vi "探头温度系数.vi"(7 "校准参数":u16(ring) caption="校准参数：" items=["pH", "DO", "浊度", "电导率", "叶绿素a", "藻密度", "ORP", "DO2", "氯化物", "悬浮物"], 8 "error in (no error)":errorcluster caption="错误输入（无错误）", 11 "温度系数":dbl=25.0 caption="温度系数：" format="%#_6f") -> (0 "error out":errorcluster caption="错误输出")   [LabVIEW 2016, in "斯坦道多参数.lvlib"]
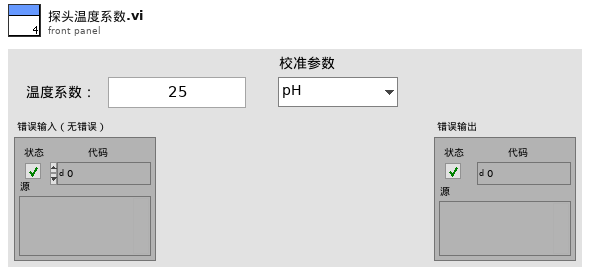
[diagram p1: front panel]
types:
  T1 = typedef "斯坦道多参数.lvlib/探头类型.ctl" = enum16{"禹山", "国弘", "纳清", "STD"}
  T2 = enum16{"NULL", "pH", "Cond", "DO", "Turb", "ORP"}
  T3 = enum16{"null", "pH", "DO", "浊度", "电导率", "叶绿素a", "藻密度"}
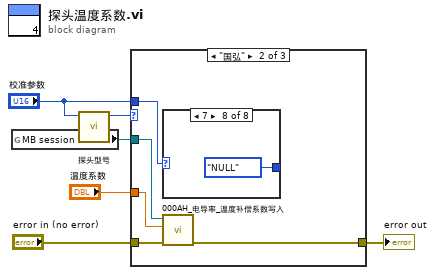
[diagram p0: block diagram]
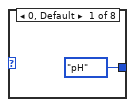
[diagram p3: hidden frame]
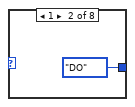
[diagram p4: hidden frame]
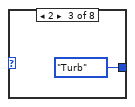
[diagram p5: hidden frame]
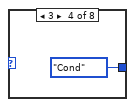
[diagram p6: hidden frame]
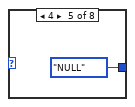
[diagram p7: hidden frame]
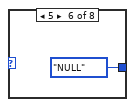
[diagram p8: hidden frame]
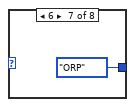
[diagram p9: hidden frame]
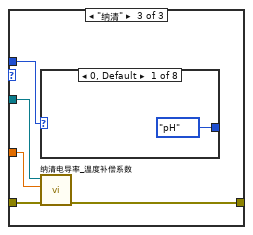
[diagram p10: hidden frame]
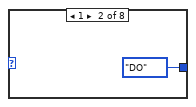
[diagram p11: hidden frame]
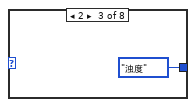
[diagram p12: hidden frame]
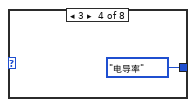
[diagram p13: hidden frame]
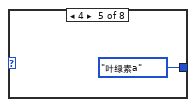
[diagram p14: hidden frame]
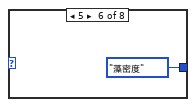
[diagram p15: hidden frame]
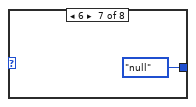
[diagram p16: hidden frame]
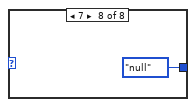
[diagram p17: hidden frame]
diagram:
  n1 = global read "多参数全局变量.vi" "MB session in"() -> (w1:refnum<class "MB_Master.lvclass">)
  n2 = call "探头型号.vi"("校准参数"="校准参数") -> ("探头型号"=w6:T1)  [unwired: 8 in, 2 out]
  n3 = case shown="\"国弘\"" w6 {
    tunnel: "校准参数" -> [_ w12 w25]
    tunnel: "error in (no error)" -> [w7 w11 w24]
    tunnel: [w7 w10 w23] -> w3
    tunnel: "温度系数" -> [_ w9 w21]
    tunnel: w1 -> [_ w8 w22]
    frame "禹山", Default {
    }
    frame "国弘" {
      n4 = case shown="7" w12 {
        tunnel: [T2."pH" ("探头") T2."DO" ("探头") T2."Turb" ("探头") T2."Cond" ("探头") T2."NULL" ("探头") T2."NULL" ("探头") T2."ORP" ("探头") T2."NULL" ("探头")] -> _
        frame 0, Default {
        }
        frame 1 {
        }
        frame 2 {
        }
        frame 3 {
        }
        frame 4 {
        }
        frame 5 {
        }
        frame 6 {
        }
        frame 7 {
        }
      }
      n5 = call "000AH_电导率_温度补偿系数写入.vi"("error in (no error)"=w11, "数值"=w9, "MB session in"=w8) -> ("error out"=w10:errorcluster)  [unwired: 7 in, 1 out]
    }
    frame "纳清" {
      n6 = case shown="0, Default" w25 {
        tunnel: [T3."pH" ("探头") T3."DO" ("探头") T3."浊度" ("探头") T3."电导率" ("探头") T3."叶绿素a" ("探头") T3."藻密度" ("探头") T3."null" ("探头") T3."null" ("探头")] -> _
        frame 0, Default {
        }
        frame 1 {
        }
        frame 2 {
        }
        frame 3 {
        }
        frame 4 {
        }
        frame 5 {
        }
        frame 6 {
        }
        frame 7 {
        }
      }
      n7 = call "纳清电导率_温度补偿系数.vi"("error in (no error)"=w24, "数值"=w21, "MB session in"=w22) -> ("error out"=w23:errorcluster)  [unwired: 7 in, 1 out]
    }
  }
  "error out" <- w3
